vi "CursorBase.vi"(8 "Enable":bool, 11 "XYGraph in":refnum<vi>) -> ()   [LabVIEW 2017]
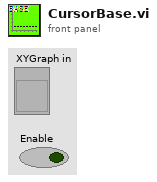
[diagram p1: front panel]
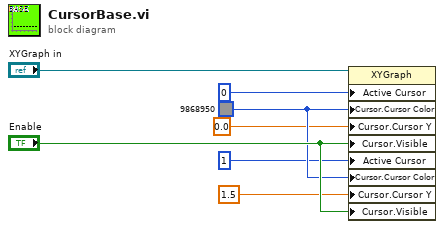
[diagram p0: block diagram]
diagram:
  w6 = u32 9868950
  n1 = property class="XYGraph"(reference="XYGraph in", "Active Cursor"=u32 0, "Cursor.Cursor Color"=w6, "Cursor.Cursor Y"=0.0 ("Cursor.Cursor Position:Cursor Y"), "Cursor.Visible"="Enable", "Active Cursor"=u32 1, "Cursor.Cursor Color"=w6, "Cursor.Cursor Y"=1.5 ("y"), "Cursor.Visible"="Enable") -> ()  [unwired: 1 in, 2 out]
